vi "set_stage (SubVI).vi"(0 "Tot Stage Arr":dbl[](array[numeric]), 1 "Volt vs pos array":cluster{dbl, dbl}[](array[cluster]), 2 "small amp":dbl=1.0 format="%0.2p", 3 "small amp freq":dbl=10.0 format="%0.2p", 4 "Add small amp?":bool, 5 "electrode arr":dbl[][](array[numeric]), 7 "signal type":T1(ring), 9 "electrodes task":refnum<k21>, 11 "electrodes task error":errorcluster, 12 "Num samples":i32, 13 "Use arb force?":bool, 14 "Electrode to sweep":i32) -> (8 "electrode_stage_arr":dbl[][](array[numeric]), 10 "electrodes task 2":refnum<k21>, 15 "electrodes task error 2":errorcluster)   [LabVIEW 2018]
uses:
  <vilib>/measure/NI_MABase.lvlib
  <resource>/objmgr/daqmx.rc
panel:
  out "Waveform Graph":dbl[][](graph)
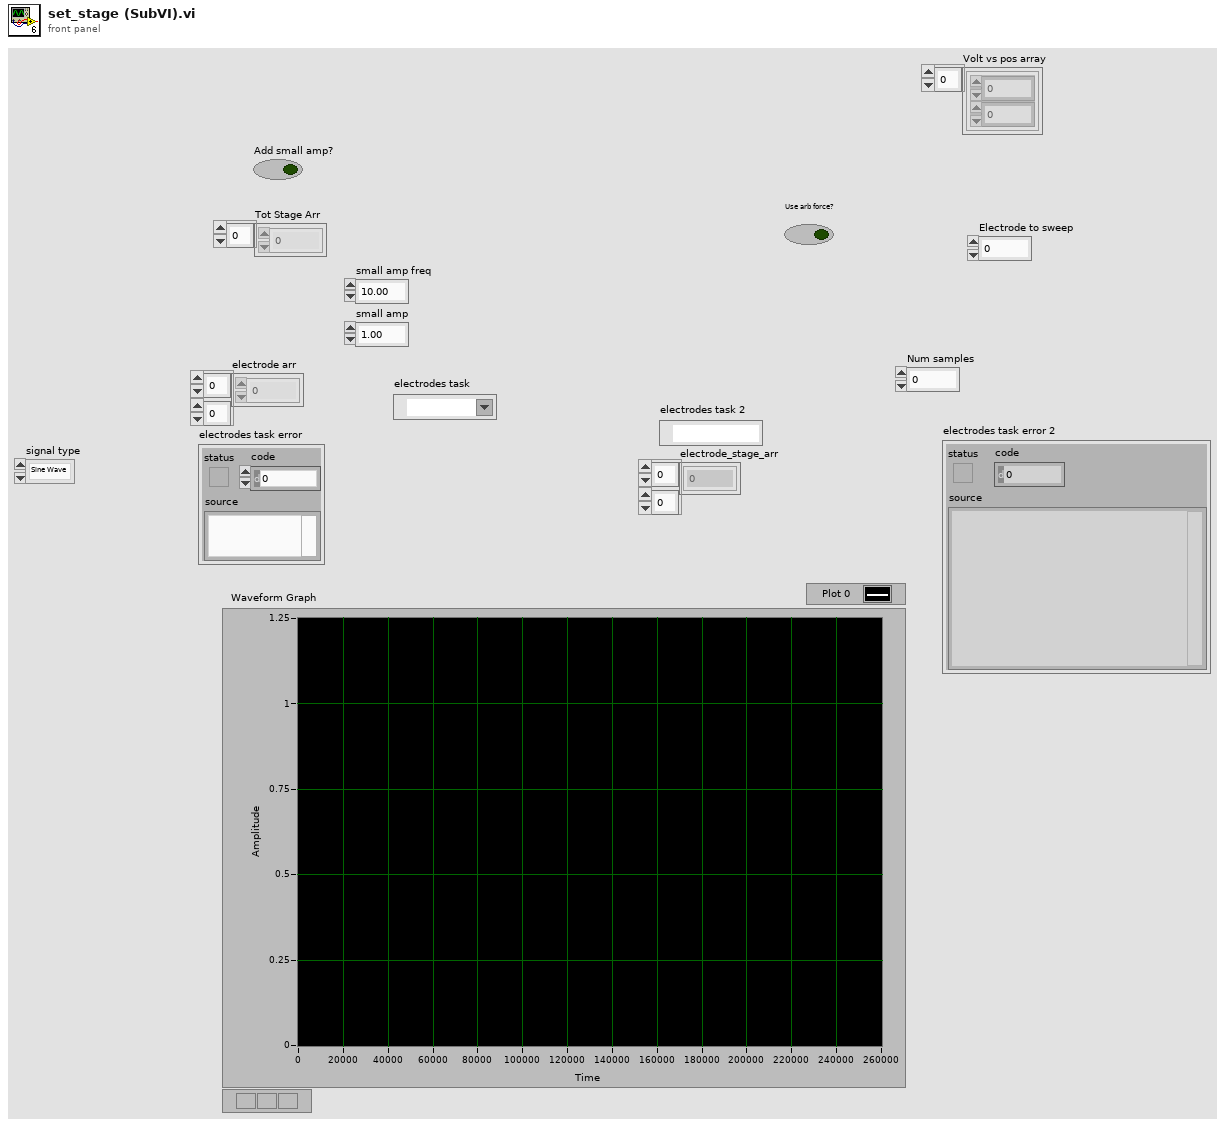
[diagram p1: front panel]
types:
  T1 = enum16{"Sine Wave", "Triangle Wave", "Square Wave", "Sawtooth Wave"}
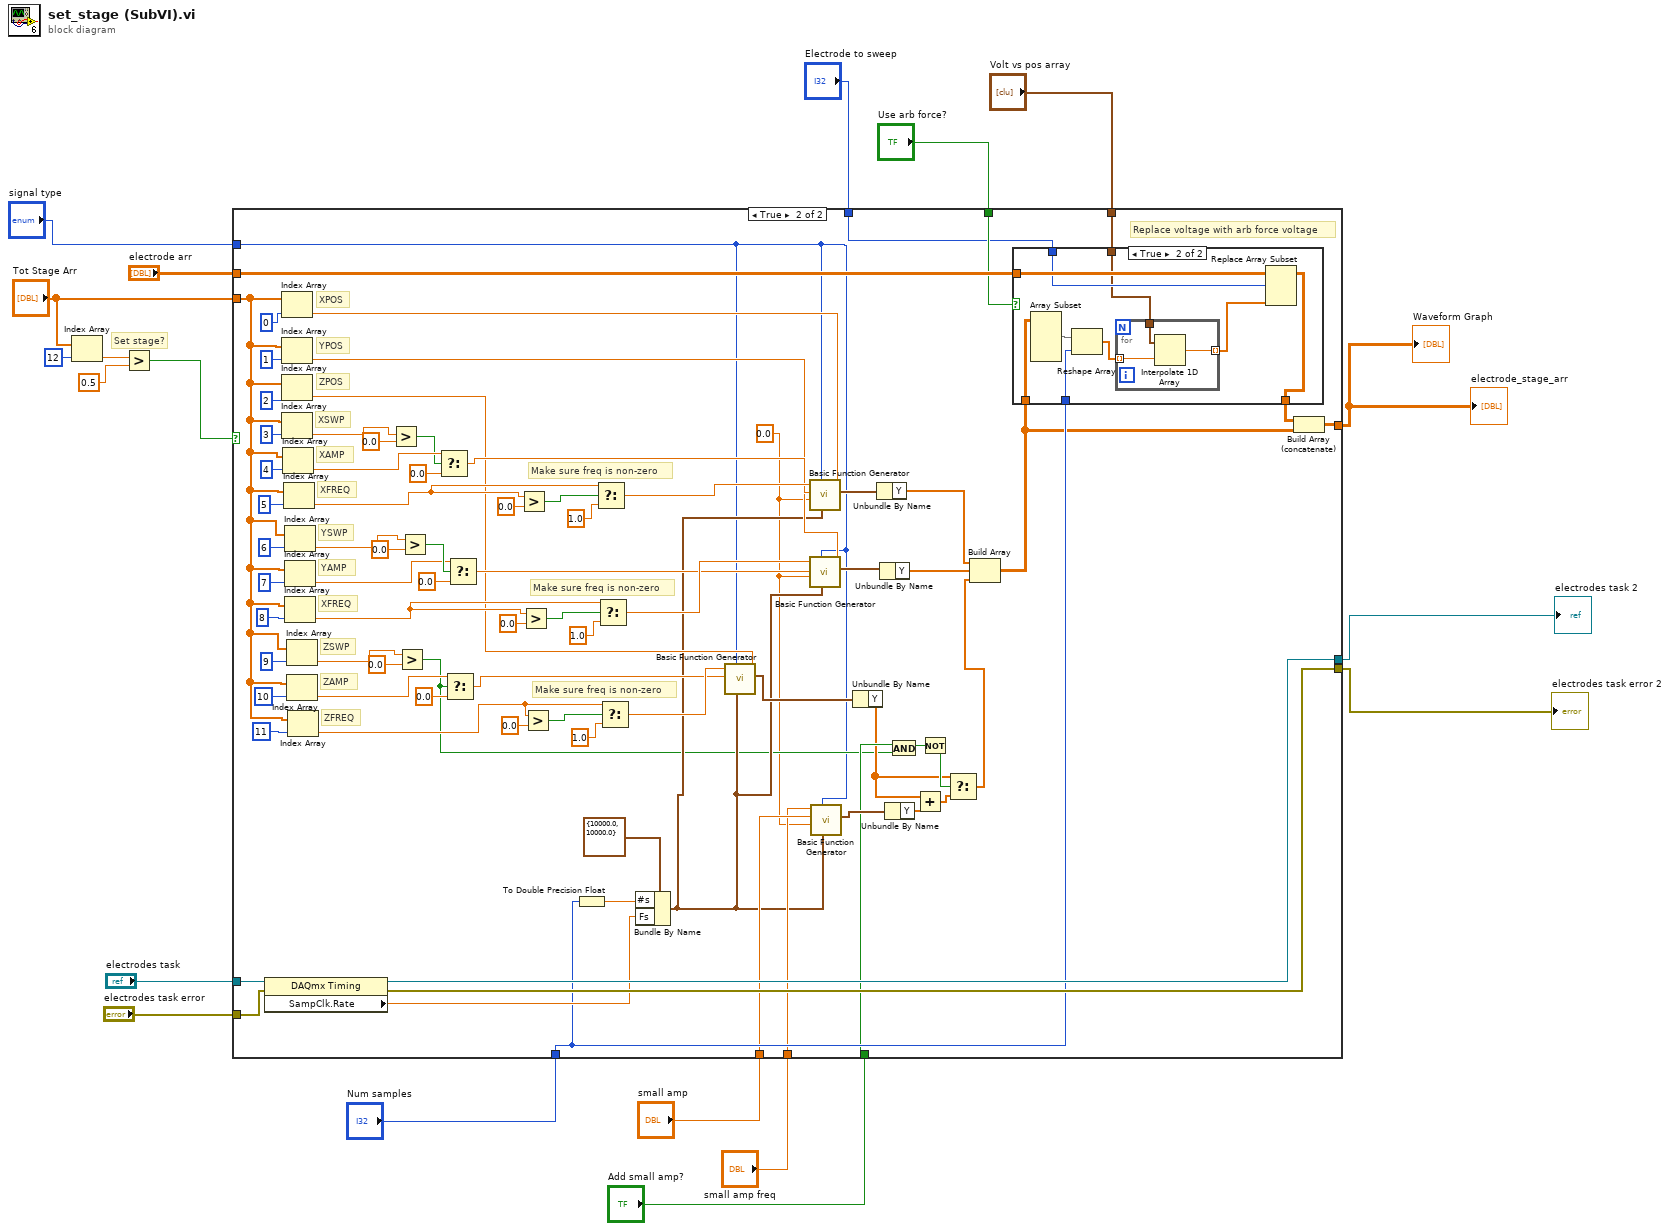
[diagram p0: block diagram]
diagram:
  # "Set stage?"
  n1 = Index Array(array="Tot Stage Arr", index=12) -> (element=w18:dbl)
  n2 = Greater?(x=w18, y=0.5) -> (0:w16:bool)
  n3 = case shown="True" w16 {
    tunnel: "electrode arr" -> [w22 w94]
    tunnel: [w22 w96] -> w11
    tunnel: "Tot Stage Arr" -> [_ w37]
    tunnel: "electrodes task" -> [w21 w102]
    tunnel: "electrodes task error" -> [w20 w101]
    tunnel: [w21 w100] -> w1
    tunnel: [w20 w99] -> w2
    tunnel: "Num samples" -> [_ w89]
    tunnel: "small amp freq" -> [_ w30]
    tunnel: "small amp" -> [_ w31]
    tunnel: "Add small amp?" -> [_ w32]
    tunnel: "Use arb force?" -> [_ w92]
    tunnel: "Electrode to sweep" -> [_ w91]
    tunnel: "Volt vs pos array" -> [_ w90]
    tunnel: "signal type" -> [_ w25]
    frame False {
    }
    frame True {
      w23 = 0.0 ("y")
      # "Make sure freq is non-zero"
      # "Make sure freq is non-zero"
      # "Make sure freq is non-zero"
      # "ZFREQ"
      # "ZAMP"
      # "ZSWP"
      # "XFREQ"
      # "YAMP"
      # "YSWP"
      # "XFREQ"
      # "XAMP"
      # "XSWP"
      # "Replace voltage with arb force voltage"
      # "ZPOS"
      # "YPOS"
      # "XPOS"
      n4 = property class="DAQmx Timing"(reference=w102, error in=w101) -> (reference out=w100:refnum<k21>, error out=w99:errorcluster, "SampClk.Rate"=w97:dbl)
      n5 = Index Array(array=w37, index=0) -> (element=w36:dbl)
      n6 = Index Array(array=w37, index=1) -> (element=w35:dbl)
      n7 = Index Array(array=w37, index=2) -> (element=w34:dbl)
      n8 = Index Array(array=w37, index=3) -> (element=w76:dbl)
      n9 = Index Array(array=w37, index=4) -> (element=w78:dbl)
      n10 = Index Array(array=w37, index=5) -> (element=w56:dbl)
      n11 = Index Array(array=w37, index=6) -> (element=w69:dbl)
      n12 = Index Array(array=w37, index=7) -> (element=w66:dbl)
      n13 = Index Array(array=w37, index=8) -> (element=w55:dbl)
      n14 = Index Array(array=w37, index=9) -> (element=w68:dbl)
      n15 = Index Array(array=w37, index=10) -> (element=w67:dbl)
      n16 = Index Array(array=w37, index=11) -> (element=w54:dbl)
      n17 = Greater?(x=w76, y=0.0) -> (0:w75:bool)
      n18 = Greater?(x=w68, y=0.0) -> (0:w26:bool)
      n19 = Greater?(x=w69, y=0.0) -> (0:w72:bool)
      n20 = Select(t=w78, s=w75, f=0.0) -> (s? t:f=w52:dbl)
      n21 = Select(t=w67, s=w26, f=0.0) -> (s? t:f=w48:dbl)
      n22 = Select(t=w66, s=w72, f=0.0) -> (s? t:f=w49:dbl)
      n23 = Greater?(x=w56, y=0.0) -> (0:w63:bool)
      n24 = Greater?(x=w55, y=0.0) -> (0:w60:bool)
      n25 = Greater?(x=w54, y=0.0) -> (0:w57:bool)
      n26 = To Double Precision Float(number=w89) -> (double precision float=w95:dbl)
      n27 = Select(t=w56, s=w63, f=1.0) -> (s? t:f=w53:dbl)
      n28 = Select(t=w55, s=w60, f=1.0) -> (s? t:f=w50:dbl)
      n29 = Select(t=w54, s=w57, f=1.0) -> (s? t:f=w51:dbl)
      n30 = Bundle By Name(cluster=cluster{"Fs":dbl, "#s":dbl} {"Fs"=10000.0, "#s"=10000.0} ("sampling info"), "#s"=w95, "Fs"=w97) -> (w29:cluster{"Fs":dbl, "#s":dbl})
      n31 = call <vilib>:"Basic Function Generator.vi"("offset"=w34, "sampling info"=w29, "signal type"=w25, "amplitude"=w48, "frequency"=w51) -> ("signal out"=w45:waveform(dbl))  [unwired: 4 in, 2 out]
      n32 = call <vilib>:"Basic Function Generator.vi"("offset"=w36, "sampling info"=w29, "signal type"=w25, "phase"=w23, "amplitude"=w52, "frequency"=w53) -> ("signal out"=w46:waveform(dbl))  [unwired: 3 in, 2 out]
      n33 = call <vilib>:"Basic Function Generator.vi"("offset"=w35, "sampling info"=w29, "signal type"=w25, "phase"=w23, "amplitude"=w49, "frequency"=w50) -> ("signal out"=w47:waveform(dbl))  [unwired: 3 in, 2 out]
      n34 = call <vilib>:"Basic Function Generator.vi"("sampling info"=w29, "signal type"=w25, "phase"=w23, "amplitude"=w31, "frequency"=w30) -> ("signal out"=w33:waveform(dbl))  [unwired: 4 in, 2 out]
      n35 = Unbundle By Name(w45) -> ("Y"=w28:dbl[])
      n36 = Unbundle By Name(w46) -> ("Y"=w44:dbl[])
      n37 = Unbundle By Name(w47) -> ("Y"=w43:dbl[])
      n38 = Unbundle By Name(w33) -> ("Y"=w41:dbl[])
      n39 = And(x=w32, y=w26) -> (x .and. y?=w38:bool)
      n40 = Add(x=w28, y=w41) -> (x+y=w40:dbl[])
      n41 = Not(x=w38) -> (.not. x?=w39:bool)
      n42 = Select(t=w28, s=w39, f=w40) -> (s? t:f=w27:dbl[])
      n43 = Build Array(w44, w43, w27) -> (w42:dbl[][])
      n44 = case shown="True" w92 {
        tunnel: w94 -> [w105 w114]
        tunnel: [w105 w113] -> w93
        tunnel: w91 -> [_ w112]
        tunnel: w42 -> [_ w111]
        tunnel: w90 -> [_ w107]
        tunnel: w89 -> [_ w106]
        frame False {
        }
        frame True {
          n45 = Array Subset(array=w111) -> (w110:dbl[][])  [unwired: 4 in]
          n46 = Reshape Array(w110, w106) -> (w109:dbl[])
          n47 = for {
            tunnel: w109 -> [w117] mode=indexing
            tunnel: [w116] -> w108 mode=indexing
            tunnel: w107 -> [w115]
            n48 = Interpolate 1D Array(1:w117, 2:w115) -> (0:w116:dbl)
          }
          n49 = Replace Array Subset(array=w114, new element=w108, index (row)=w112) -> (w113:dbl[][])  [unwired: 1 in]
        }
      }
      n50 = Build Array (concatenate)(w93, w42) -> (w96:dbl[][])
    }
  }
  "electrodes task 2" <- w1
  "electrodes task error 2" <- w2
  "Waveform Graph" <- w11
  "electrode_stage_arr" <- w11
